vi "Finite Generation.vi"() -> ()   [LabVIEW 2021, in "GettingStarted_5745_Host.lvlib"]
uses:
  GettingStarted_5745_Host.lvlib
  <vilib>/userdefined/High Color/nirio_resource_hc.ctl
  <instrlib>/FlexRIO/API/Host/v1/NI FlexRIO/API/Reference Clock Source.ctl
  <vilib>/rvi/interface/common/niFpgaWaitOnOcc.vi
  <vilib>/Utility/error.llb/Error Cluster From Error Code.vi
  <instrlib>/FlexRIO/API/Host/v1/NI FlexRIO/API/Configure Reference Clock.vi
  <instrlib>/FlexRIO/API/Host/v1/NI FlexRIO/API/Configure Immediate Start Trigger.vi
  <instrlib>/_niInstr/Streaming/v1/Host/Public/Start Finite Stream.vi
  <vilib>/FPGAPlugInAG/Dynamic/niLvFpga_Close_Dynamic.vi
  <vilib>/rvi/interface/nirviMethod/nirviMethod.xnode
  <vilib>/rvi/interface/nirviCloseFPGA/nirviCloseFPGA.xnode
  <instrlib>/FlexRIO/API/Host/v1/NI FlexRIO API v1.lvlib
  <instrlib>/_niInstr/Streaming/v1/Host/niInstr Streaming v1 Host.lvlib
  <vilib>/FPGAPlugInAG/Dynamic/niLvFpga_ConfigureFifo_Dynamic.vi
  <vilib>/rvi/errors/niLvFpgaMergeErrorWithErrorCode.vi
panel:
  in  "Amplitude (V) AO1":dbl=0.4 format="%0.2p"
  in  "Amplitude (V) AO0":dbl=0.4 format="%0.2p"
  in  "signal type AO1":T1(ring)
  in  "signal type AO0":T1(ring)
  in  "Send Signal":bool caption="Download AO Waveforms"
  out "AO Out":waveform(dbl)[](graph) caption="Waveform Graph"
  in  "stop":bool
  in  "Bitfile path":path=path "C:/Program Files (x86)/National Instruments/LabVIEW 2022/ProjectTemplates/Source/FlexRIO/NI5745/Getting Started/FPGA Bitfiles/PXIe_5745_KU040.lvbitx"
  out "error out":errorcluster
  in  "RIO Device":T2="5745_1"
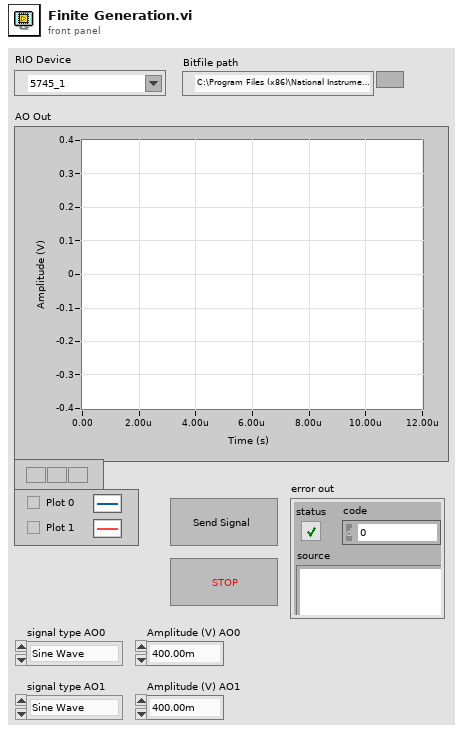
[diagram p1: front panel]
types:
  T1 = enum16{"Sine Wave", "Triangle Wave", "Square Wave", "Sawtooth Wave"}
  T2 = typedef "nirio_resource_hc.ctl" = tag
  T3 = typedef "NI FlexRIO API v1.lvlib/Reference Clock Source.ctl" = i32
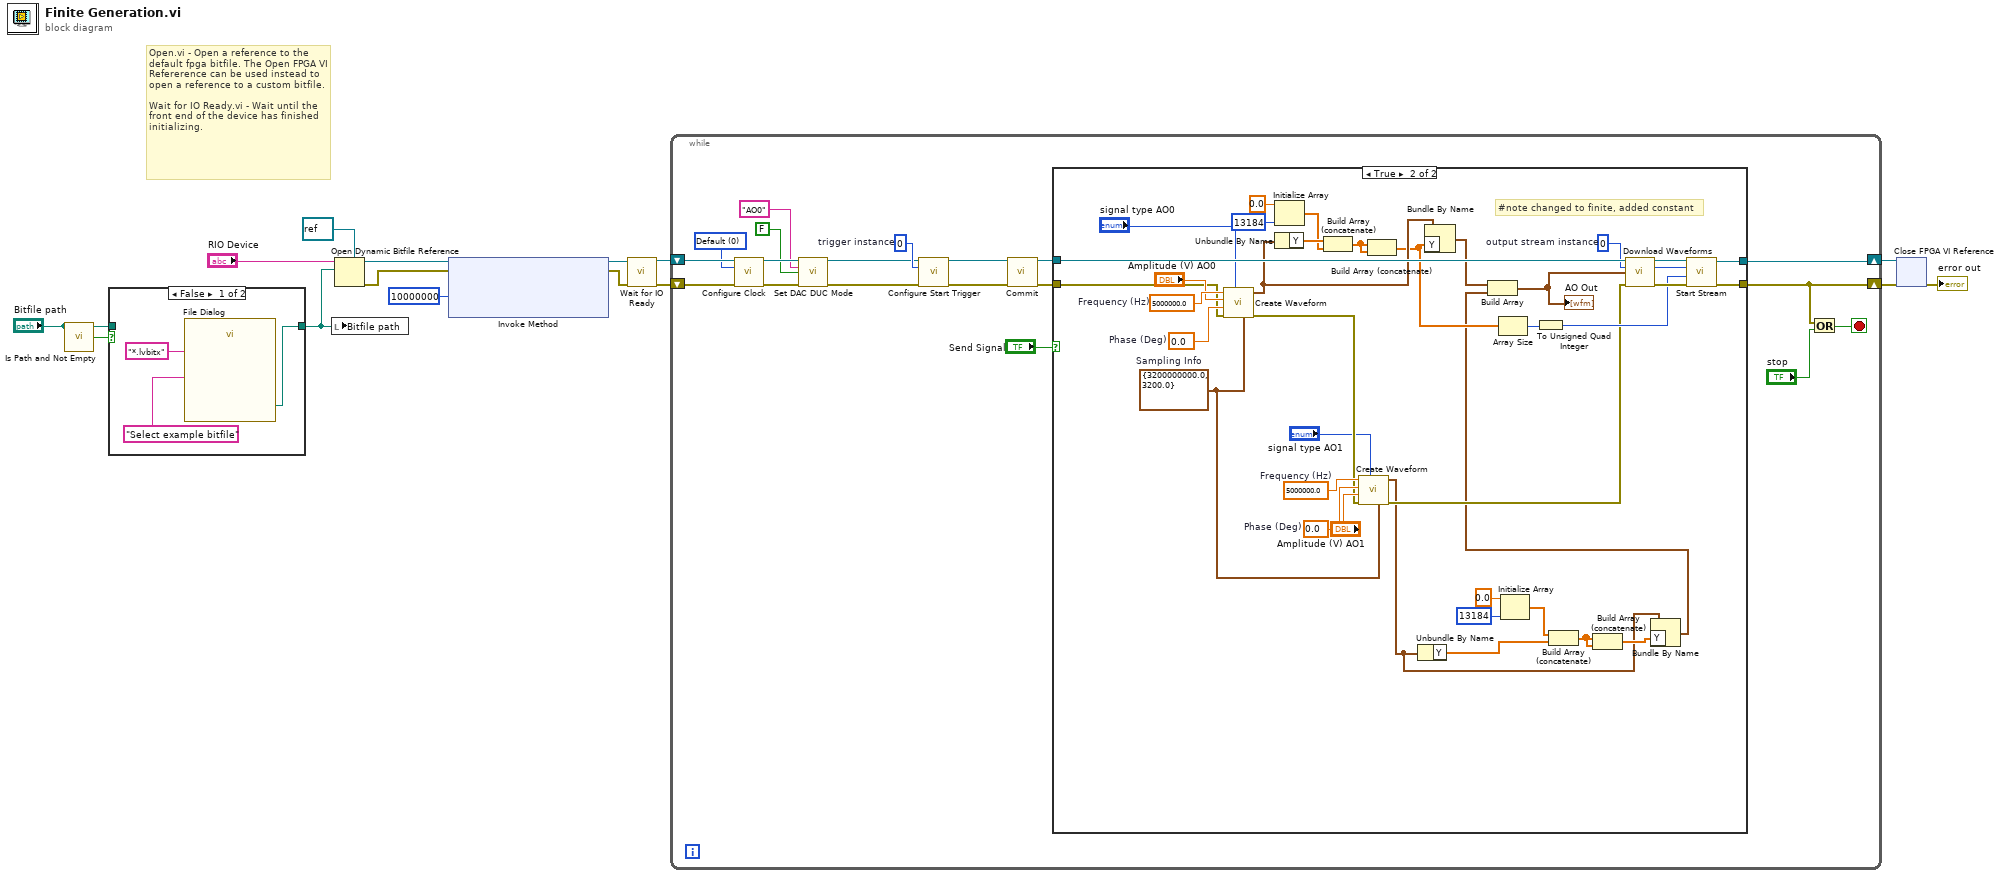
[diagram p0: block diagram]
diagram:
  # "Open.vi - Open a reference to the default fpga bitfile. The Open FPGA VI Refererence can be used instead to open a reference to a custom bitfile.\n\nWait for IO Ready.vi - Wait until the front end of the device has finished initializing."
  n1 = call <vilib>:"Is Path and Not Empty.vi"("path"="Bitfile path") -> ("Is Path and Not Empty?"=w7:bool)  [unwired: 4 in]
  n2 = case shown="False" w7 {
    tunnel: "Bitfile path" -> [_ w19]
    tunnel: [w17 w19] -> w6
    frame False {
      n3 = call "File Dialog"("prompt"="Select example bitfile", "pattern (all files)"="*.lvbitx") -> ("selected path"=w17:path)  [unwired: 10 in, 3 out]
    }
    frame True {
    }
  }
  n4 = local write "Bitfile path"(w6) -> ()
  n5 = Open Dynamic Bitfile Reference(0:"RIO Device", 1:w6, 4:refnum<k20> refnum ("Type")) -> (5:w12:refnum<k20>, 8:w3:errorcluster)  [unwired: 2 in]
  n6 = xnode "Invoke Method"("FPGA VI Reference In"=w12, "error in"=w3, "Requested Depth"=u32 10000000) -> ("FPGA VI Reference Out"=w5:refnum<k20>, "error out"=w2:errorcluster)  [unwired: 1 out]
  n7 = call <instrlib>:"Wait for IO Ready.vi"("fpga interface in"=w5, "error in"=w2) -> ("fpga interface out"=w13:refnum<k20>, "error out"=w14:errorcluster)  [unwired: 10 in, 2 out]
  n8 = while {
    shift-right: [w28] -> w9
    shift-left: w14 -> [w35]
    shift-right: [w29] -> w10
    shift-left: w13 -> [w34]
    stop <- w25 stop-if-true
    w20 = T3 0 items=["Default", "Onboard", "PXI_Clk10", "External", "None", "Baseboard Reference"] ("reference clock source")
    w36 = u32 0  # trigger instance
    n9 = call-poly <instrlib>:"Configure Clock.vi"("fpga interface in"=w34, "reference clock source"=w20, "error in"=w35) -> ("fpga interface out"=w38:refnum<k20>, "error out"=w37:errorcluster)  [unwired: 11 in]
    n10 = call "Set DAC DUC Mode.vi"("fpga interface in"=w38, "DAC Digital Upconverter Channel"="AO0", "Enable DAC Digital Upconverter"=FALSE, "error in (no error)"=w37) -> ("fpga interface out"=w22:refnum<k20>, "error out"=w23:errorcluster)  [unwired: 10 in]
    n11 = call-poly <instrlib>:"Configure Start Trigger.vi"("fpga interface in"=w22, "trigger instance"=w36, "error in"=w23) -> ("fpga interface out"=w32:refnum<k20>, "error out"=w31:errorcluster)  [unwired: 10 in, 1 out]
    n12 = call <instrlib>:"Commit.vi"("fpga interface in"=w32, "error in"=w31) -> ("fpga interface out"=w33:refnum<k20>, "error out"=w27:errorcluster)  [unwired: 12 in]
    n13 = case shown="True" "Send Signal" {
      tunnel: w33 -> [w40 w74]
      tunnel: [w40 w69] -> w29
      tunnel: [w39 w68] -> w28
      tunnel: w27 -> [w39 w67]
      frame False {
      }
      frame True {
        w54 = 5000000.0  # Frequency (Hz)
        w56 = 0.0  # Phase (Deg)
        w76 = 5000000.0  # Frequency (Hz)
        w50 = cluster{"Fs":dbl, "#s":dbl} {"Fs"=3200000000.0, "#s"=3200.0}  # Sampling Info
        w73 = 0.0  # Phase (Deg)
        w72 = 0  # output stream instance
        # "#note changed to finite, added constant"
        n14 = call "Create Waveform.vi"("sampling info"=w50, "signal type"="signal type AO0", "error in (no error)"=w67, "phase"=w73, "amplitude"="Amplitude (V) AO0", "frequency"=w76) -> ("error out"=w53:errorcluster, "Output Waveform (V)"=w63:waveform(dbl))  [unwired: 3 in, 1 out]
        n15 = Initialize Array(0.0 ("element"), 13184 ("dimension size")) -> (w62:dbl[])
        n16 = Unbundle By Name(w63) -> ("Y"=w64:dbl[])
        n17 = Build Array (concatenate)(w64, w62) -> (w58:dbl[])
        n18 = call "Create Waveform.vi"("sampling info"=w50, "signal type"="signal type AO1", "error in (no error)"=w53, "phase"=w56, "amplitude"="Amplitude (V) AO1", "frequency"=w54) -> ("error out"=w52:errorcluster, "Output Waveform (V)"=w43:waveform(dbl))  [unwired: 3 in, 1 out]
        n19 = Build Array (concatenate)(w58, w58) -> (w59:dbl[])
        n20 = Unbundle By Name(w43) -> ("Y"=w46:dbl[])
        n21 = Bundle By Name(cluster=w63, "Y"=w59) -> (w57:waveform(dbl))
        n22 = Array Size(array=w59) -> (size(s)=w61:i32)
        n23 = Initialize Array(0.0 ("element"), 13184 ("dimension size")) -> (w47:dbl[])
        n24 = To Unsigned Quad Integer(1:w61) -> (0:w60:u64)
        n25 = Build Array (concatenate)(w47, w46) -> (w49:dbl[])
        n26 = Build Array (concatenate)(w49, w49) -> (w48:dbl[])
        n27 = Bundle By Name(cluster=w43, "Y"=w48) -> (w42:waveform(dbl))
        n28 = Build Array(w57, w42) -> (w70:waveform(dbl)[])
        "AO Out" <- w70
        n29 = call "Download Waveforms.vi"("fpga interface in"=w74, "stream instance"=w72, "waveforms"=w70, "error in"=w52) -> ("fpga interface out"=w78:refnum<k20>, "stream instance out"=w71:i32, "error out"=w77:errorcluster)  [unwired: 9 in]
        n30 = call-poly <instrlib>:"Start Stream.vi"("error in (no error)"=w77, "num samples"=w60, "stream index"=w71, "refnum in"=w78) -> ("error out"=w68:errorcluster, "refnum out"=w69:refnum<k20>)  [unwired: 6 in]
      }
    }
    n31 = Or(x=w28, y="stop") -> (x .or. y?=w25:bool)
  }
  n32 = xnode "Close FPGA VI Reference"("FPGA VI Reference In"=w10, "error in"=w9) -> ("error out"=→"error out":errorcluster)
